vi "daemon.vi"(8 "error in (no error)":errorcluster, 10 "callback notifier":refnum<notifier>, 11 "EventDaemon.lvclass":refnum<class "TemplateDaemon.lvclass">) -> (0 "error out":errorcluster)   [LabVIEW 2024, in "TemplateDaemon.lvclass"]
doc: "Main daemon loop for class. Uses public access to start, stop and handle event-based messages."
uses:
  TemplateDaemon.lvclass
  status--cluster.ctl
  states--enum.ctl
  TemplateDaemon.lvclass/TemplateDaemon.ctl
panel:
  out "status":T1
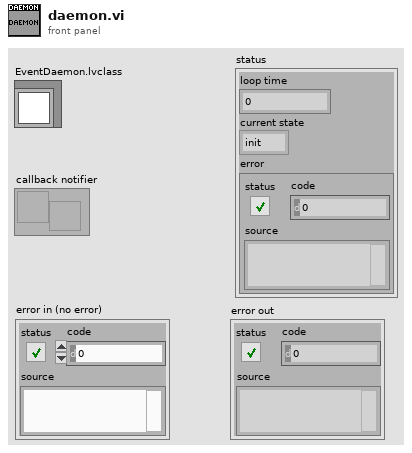
[diagram p1: front panel]
types:
  T1 = typedef "TemplateDaemon.lvclass/status--cluster.ctl" = cluster{"loop time":u32, "current state":T2, "error":errorcluster}
  T2 = typedef "TemplateDaemon.lvclass/states--enum.ctl" = enum16{"init", "default", "error handler", "exit"}
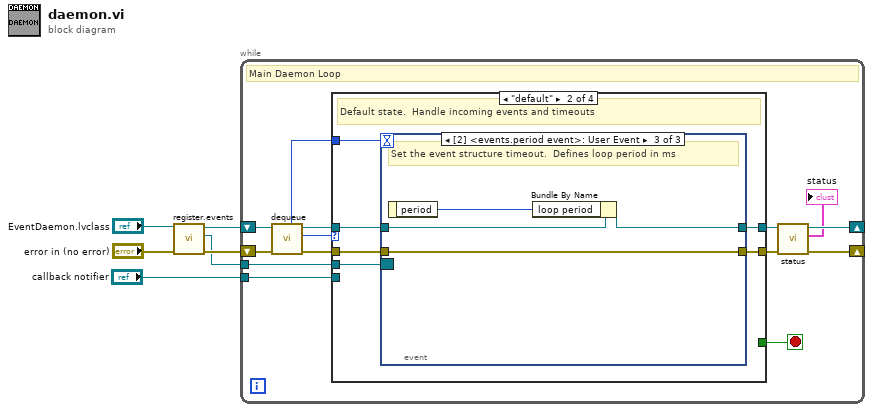
[diagram p0: block diagram]
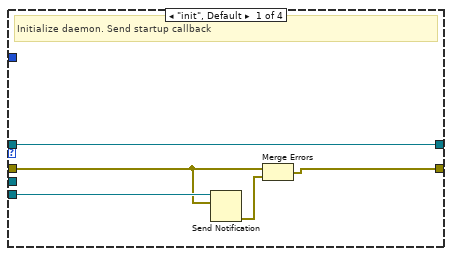
[diagram p2: hidden frame]
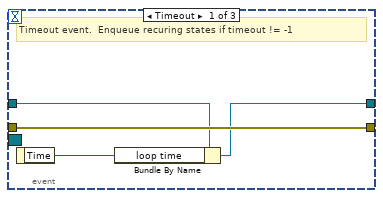
[diagram p3: hidden frame]
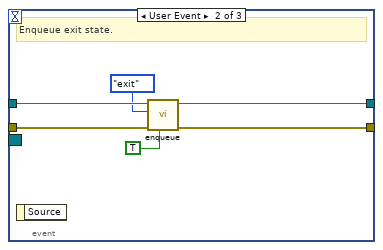
[diagram p4: hidden frame]
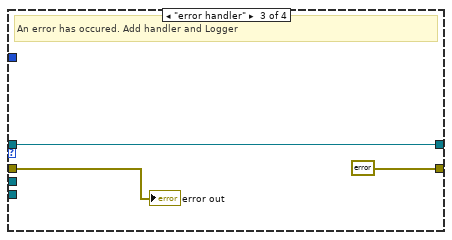
[diagram p5: hidden frame]
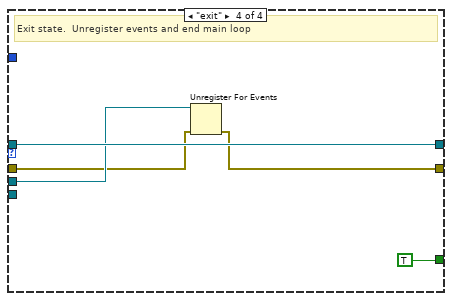
[diagram p6: hidden frame]
diagram:
  n1 = call "register.events.vi"("error in (no error)"="error in (no error)", "EventDaemon in"="EventDaemon.lvclass") -> ("error out"=w4:errorcluster, "Event Registration Refnum"=w2:refnum<event-registration>, "EventDaemon out"=w3:refnum<class "TemplateDaemon.lvclass">)  [unwired: 7 in]
  n2 = while {
    shift-right: [w9] -> _
    shift-left: w4 -> [w19]
    tunnel: w2 -> [w15]
    shift-right: [w10] -> _
    shift-left: w3 -> [w20]
    tunnel: "callback notifier" -> [w7]
    stop <- w13 stop-if-true
    # "Main Daemon Loop"
    n3 = call "dequeue.vi"("error in (no error)"=w19, "EventDaemon in"=w20) -> ("error out"=w17:errorcluster, "state"=w18:T2, "EventDaemon out"=w16:refnum<class "TemplateDaemon.lvclass">, "timeout"=w14:i32)  [unwired: 6 in]
    n4 = case shown="\"default\"" w18 {
      tunnel: w17 -> [w23 w31 w48 w50]
      tunnel: w16 -> [w25 w29 w47 w52]
      tunnel: w15 -> [_ w30 _ w51]
      tunnel: w14 -> [_ w28 _ _]
      tunnel: [w25 w27 w47 w52] -> w12
      tunnel: [w21 w26 errorcluster {"status"=FALSE, "code"=0, "source"=""} ("error out") w49] -> w11
      tunnel: [_ _ _ TRUE] -> w13
      tunnel: w7 -> [w24 _ _ _]
      frame "init", Default {
        # "Initialize daemon. Send startup callback"
        n5 = Send Notification(notification=w23, notifier=w24) -> (error out=w22:errorcluster)  [unwired: 1 in, 1 out]
        n6 = Merge Errors(w23, w22) -> (w21:errorcluster)
      }
      frame "default" {
        # "Default state.  Handle incoming events and timeouts"
        n7 = event shown="[2] <events.period event>: User Event" {
          selector: w30 -> [_ _ _]
          dyn-events: _ -> [_ _ _]
          timeout: w28 -> [_ _ _]
          tunnel: w31 -> [w35 w40 w44]
          tunnel: w29 -> [w34 w41 w45]
          tunnel: [w32 w37 w42] -> w27
          tunnel: [w35 w38 w44] -> w26
          event Timeout {
            # "Timeout event.  Enqueue recuring states if timeout != -1"
            n8 = event-data() -> ("Time"=w33:u32)  [unwired: 1 in]
            n9 = Bundle By Name(cluster=w34, "loop time"=w33) -> (w32:refnum<class "TemplateDaemon.lvclass">)
          }
          event User Event {
            # "Enqueue exit state."
            n10 = event-data() -> ()  [unwired: 1 in, 1 out]
            n11 = call "enqueue.vi"("priority (f)"=TRUE ("priority"), "error in (no error)"=w40, "states"=states--enum."exit", "EventDaemon in"=w41) -> ("error out"=w38:errorcluster, "EventDaemon out"=w37:refnum<class "TemplateDaemon.lvclass">)  [unwired: 6 in]
          }
          event User Event {
            # "Set the event structure timeout.  Defines loop period in ms"
            n12 = event-data() -> ("period"=w43:i32)  [unwired: 1 in]
            n13 = Bundle By Name(cluster=w45, "loop period"=w43) -> (w42:refnum<class "TemplateDaemon.lvclass">)
          }
        }
      }
      frame "error handler" {
        # "An error has occured. Add handler and Logger"
        "error out" <- w48
      }
      frame "exit" {
        # "Exit state.  Unregister events and end main loop"
        n14 = Unregister For Events(event registration refnum=w51, error in=w50) -> (error out=w49:errorcluster)
      }
    }
    n15 = call "status.vi"("error in (no error)"=w11, "EventDaemon in"=w12) -> ("error out"=w9:errorcluster, "status"=→"status":T1, "EventDaemon out"=w10:refnum<class "TemplateDaemon.lvclass">)  [unwired: 7 in]
  }
